vi "IECMemory.Tables2Array.vi"(5 "Timing Num":dbl[](array[numeric]), 9 "Logic":string[](array[string]), 11 "error in (no error)":errorcluster) -> (8 "MemData":dbl[][](array[numeric]), 15 "error out":errorcluster)   [LabVIEW 2014, in "IECMemory.lvlib"]
uses:
  IECMemory.lvlib
panel:
  in  "Channel":i32
  in  "Index":i32
  in  "Upper/Lower?":string
  out "Decomposed Logic Strings":string[][](array[string])
  out "Logic Strings Length":i32[](array[numeric])
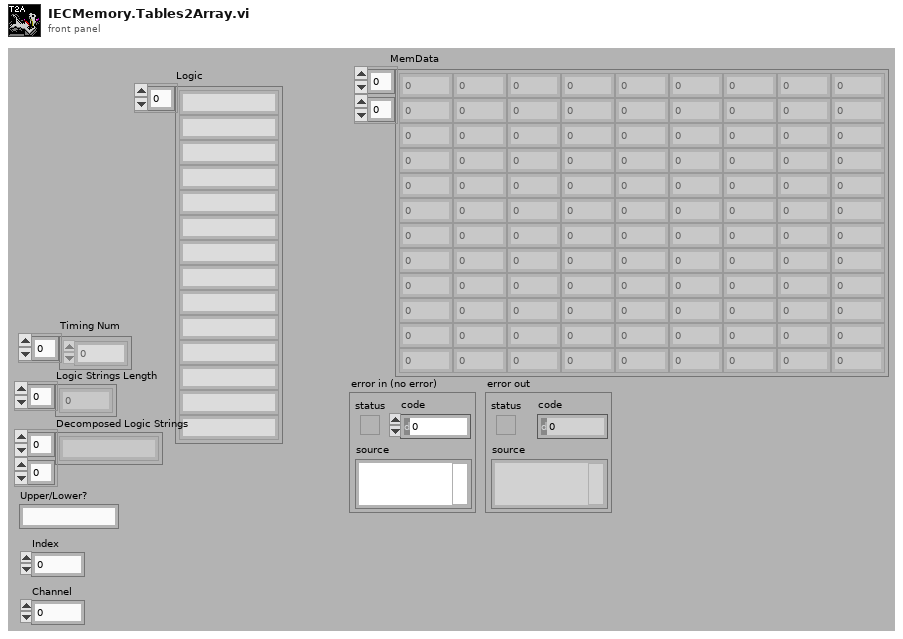
[diagram p1: front panel]
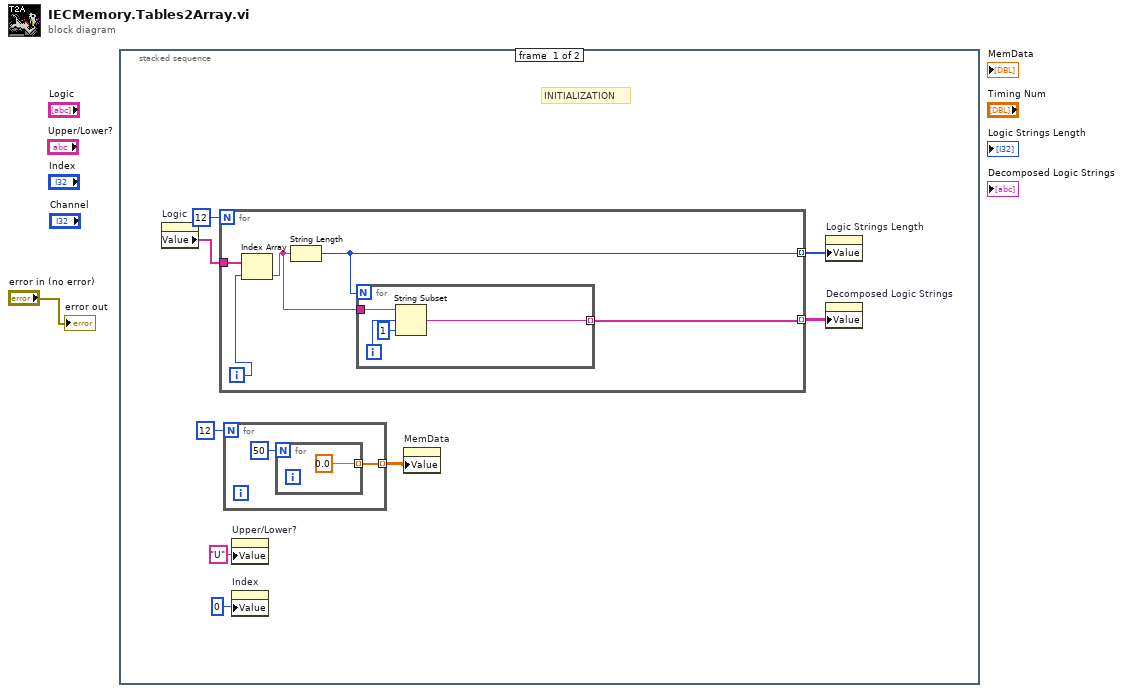
[diagram p0: block diagram]
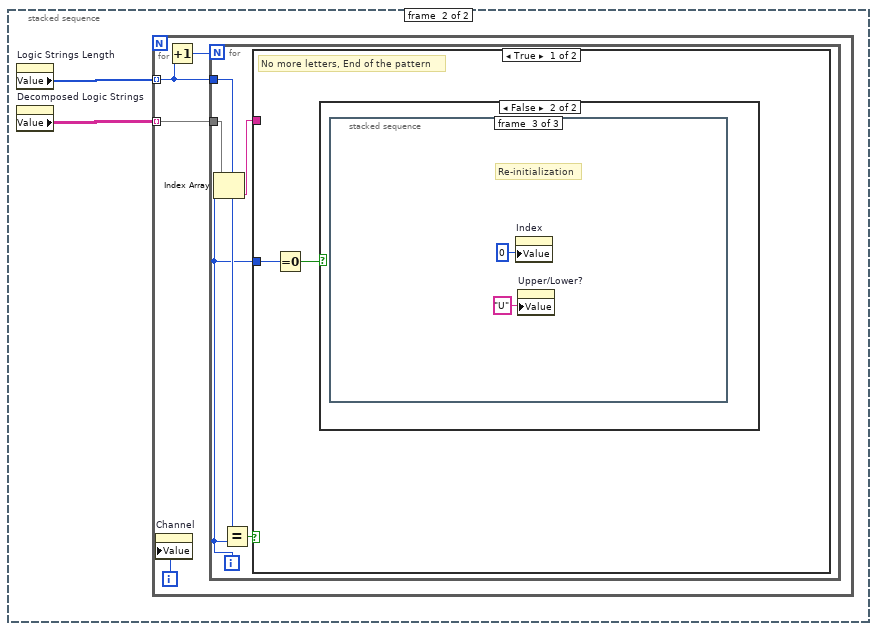
[diagram p2: hidden frame]
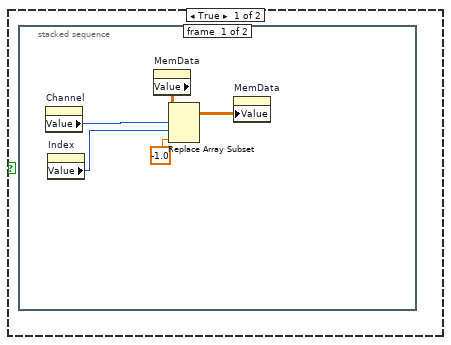
[diagram p3: hidden frame]
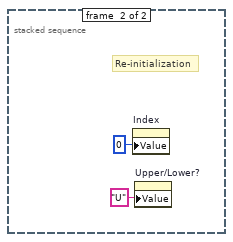
[diagram p4: hidden frame]
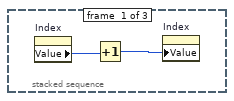
[diagram p5: hidden frame]
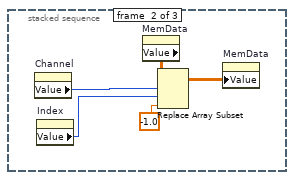
[diagram p6: hidden frame]
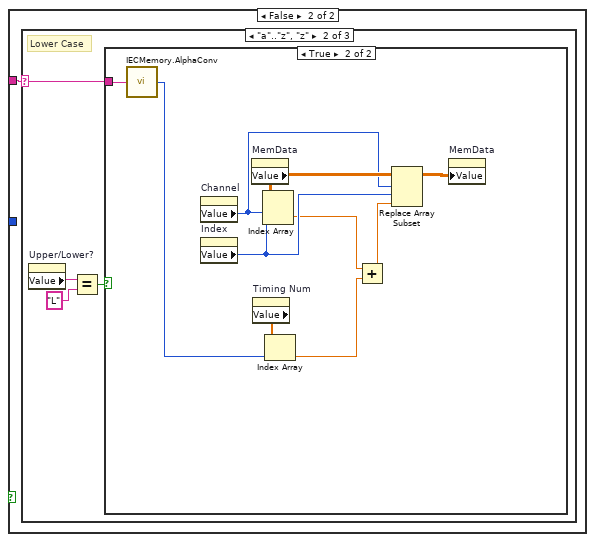
[diagram p7: hidden frame]
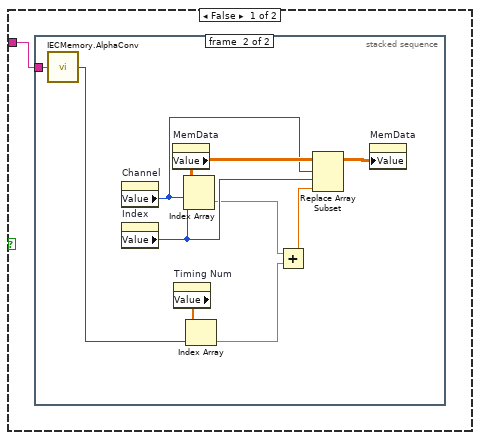
[diagram p9: hidden frame]
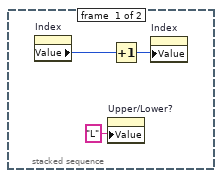
[diagram p10: hidden frame]
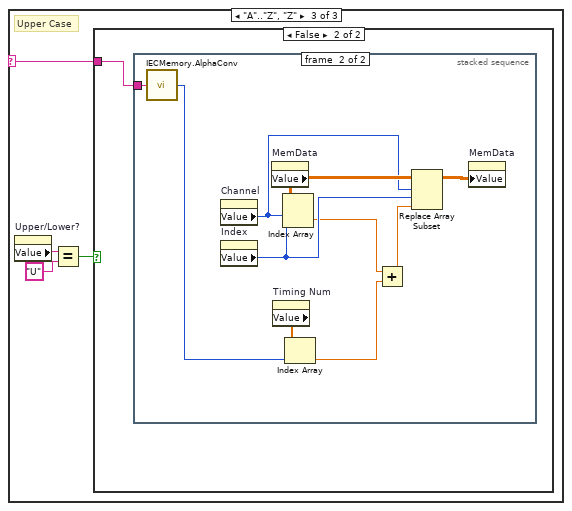
[diagram p11: hidden frame]
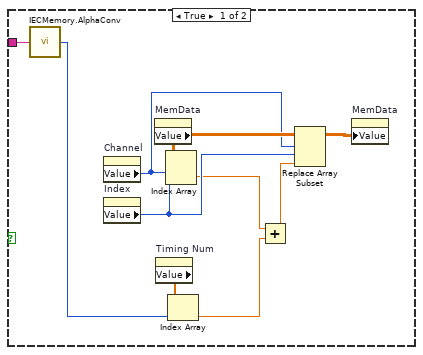
[diagram p12: hidden frame]
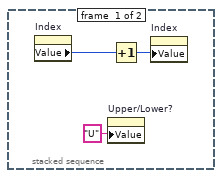
[diagram p13: hidden frame]
diagram:
  n1 = stacked-sequence {
    frame #0 {
      # "INITIALIZATION"
      n2 = property on="Logic" class="Arr (strict)"() -> ("Value"=w3:string[])  [unwired: 2 in, 2 out]
      n3 = for {
        N: 12 -> [_]
        tunnel: [w17] -> w9 mode=indexing
        tunnel: [w16] -> w8 mode=indexing
        tunnel: w3 -> [w14]
        i -> [w15]
        n4 = Index Array(array=w14, index=w15) -> (element=w13:string)
        n5 = String Length(string=w13) -> (length=w17:i32)
        n6 = for {
          N: w17 -> [_]
          tunnel: w13 -> [w21]
          tunnel: [w18] -> w16 mode=indexing
          i -> [w19]
          n7 = String Subset(string=w21, offset (0)=w19, length (rest)=1 ("length (rest)")) -> (substring=w18:string)
        }
      }
      n8 = for {
        N: 12 -> [_]
        tunnel: [w10] -> w6 mode=indexing
        n9 = for {
          N: 50 -> [_]
          tunnel: [0.0] -> w10 mode=indexing
        }
      }
      n10 = property on="Upper/Lower?" class="Str"("Value"="U" ("Upper/Lower?")) -> ()  [unwired: 2 in, 2 out]
      n11 = property on="Index" class="DigNum (strict)"("Value"=0 ("Index")) -> ()  [unwired: 2 in, 2 out]
      n12 = property on="MemData" class="Arr (strict)"("Value"=w6) -> ()  [unwired: 2 in, 2 out]
      n13 = property on="Logic Strings Length" class="Arr (strict)"("Value"=w9) -> ()  [unwired: 2 in, 2 out]
      n14 = property on="Decomposed Logic Strings" class="Arr (strict)"("Value"=w8) -> ()  [unwired: 2 in, 2 out]
    }
    frame #1 {
      n15 = property on="Logic Strings Length" class="Arr (strict)"() -> ("Value"=w22:i32[])  [unwired: 2 in, 2 out]
      n16 = property on="Decomposed Logic Strings" class="Arr (strict)"() -> ("Value"=w23:string[][])  [unwired: 2 in, 2 out]
      n17 = for {
        tunnel: w23 -> [w24] mode=indexing
        tunnel: w22 -> [w25] mode=indexing
        i -> [w27]
        n18 = property on="Channel" class="DigNum (strict)"("Value"=w27) -> ()  [unwired: 2 in, 2 out]
        n19 = Increment(x=w25) -> (x+1=w26:i32)
        n20 = for {
          N: w26 -> [_]
          tunnel: w25 -> [w32]
          tunnel: w24 -> [w30]
          i -> [w28]
          n21 = Index Array(array=w30, index=w28) -> (element=w29:string)
          n22 = Equal?(x=w32, y=w28) -> (x = y?=w31:bool)
          n23 = case shown="True" w31 {
            tunnel: w29 -> [_ w51]
            tunnel: w28 -> [w34 _]
            frame True {
              # "No more letters, End of the pattern"
              n24 = Equal To 0?(x=w34) -> (x = 0?=w33:bool)
              n25 = case shown="False" w33 {
                frame True {
                  n26 = stacked-sequence {
                    frame #0 {
                      n27 = property on="Channel" class="DigNum (strict)"() -> ("Value"=w37:i32)  [unwired: 2 in, 2 out]
                      n28 = property on="Index" class="DigNum (strict)"() -> ("Value"=w35:i32)  [unwired: 2 in, 2 out]
                      n29 = property on="MemData" class="Arr (strict)"() -> ("Value"=w39:dbl[][])  [unwired: 2 in, 2 out]
                      n30 = Replace Array Subset(array=w39, new element=-1.0, index (row)=w37, index (col)=w35) -> (w36:dbl[][])
                      n31 = property on="MemData" class="Arr (strict)"("Value"=w36) -> ()  [unwired: 2 in, 2 out]
                    }
                    frame #1 {
                      # "Re-initialization"
                      n32 = property on="Index" class="DigNum (strict)"("Value"=0 ("Index")) -> ()  [unwired: 2 in, 2 out]
                      n33 = property on="Upper/Lower?" class="Str"("Value"="U" ("Upper/Lower?")) -> ()  [unwired: 2 in, 2 out]
                    }
                  }
                }
                frame False {
                  n34 = stacked-sequence {
                    frame #0 {
                      n35 = property on="Index" class="DigNum (strict)"() -> ("Value"=w43:i32)  [unwired: 2 in, 2 out]
                      n36 = Increment(x=w43) -> (x+1=w42:i32)
                      n37 = property on="Index" class="DigNum (strict)"("Value"=w42) -> ()  [unwired: 2 in, 2 out]
                    }
                    frame #1 {
                      n38 = property on="Channel" class="DigNum (strict)"() -> ("Value"=w46:i32)  [unwired: 2 in, 2 out]
                      n39 = property on="Index" class="DigNum (strict)"() -> ("Value"=w44:i32)  [unwired: 2 in, 2 out]
                      n40 = property on="MemData" class="Arr (strict)"() -> ("Value"=w48:dbl[][])  [unwired: 2 in, 2 out]
                      n41 = Replace Array Subset(array=w48, new element=-1.0, index (row)=w46, index (col)=w44) -> (w45:dbl[][])
                      n42 = property on="MemData" class="Arr (strict)"("Value"=w45) -> ()  [unwired: 2 in, 2 out]
                    }
                    frame #2 {
                      # "Re-initialization"
                      n43 = property on="Index" class="DigNum (strict)"("Value"=0 ("Index")) -> ()  [unwired: 2 in, 2 out]
                      n44 = property on="Upper/Lower?" class="Str"("Value"="U" ("Upper/Lower?")) -> ()  [unwired: 2 in, 2 out]
                    }
                  }
                }
              }
            }
            frame False {
              n45 = case shown="\"a\"..\"z\", \"z\"" w51 {
                selector: w51 -> [_ w52 w80]
                frame "", "*", Default {
                  # "DO NOTHING"
                  # "Channel not in use"
                }
                frame "a".."z", "z" {
                  # "Lower Case"
                  n46 = property on="Upper/Lower?" class="Str"() -> ("Value"=w54:string)  [unwired: 2 in, 2 out]
                  n47 = Equal?(x=w54, y="L") -> (x = y?=w55:bool)
                  n48 = case shown="True" w55 {
                    tunnel: w52 -> [w56 w70]
                    frame False {
                      n49 = stacked-sequence {
                        tunnel: w56 -> [_ w69]
                        frame #0 {
                          n50 = property on="Index" class="DigNum (strict)"() -> ("Value"=w58:i32)  [unwired: 2 in, 2 out]
                          n51 = property on="Upper/Lower?" class="Str"("Value"="L" ("Upper/Lower?")) -> ()  [unwired: 2 in, 2 out]
                          n52 = Increment(x=w58) -> (x+1=w59:i32)
                          n53 = property on="Index" class="DigNum (strict)"("Value"=w59) -> ()  [unwired: 2 in, 2 out]
                        }
                        frame #1 {
                          n54 = call "IECMemory.AlphaConv.vi"("String"=w69) -> ("Numeric"=w64:i32)  [unwired: 14 in]
                          n55 = property on="Channel" class="DigNum (strict)"() -> ("Value"=w65:i32)  [unwired: 2 in, 2 out]
                          n56 = property on="Index" class="DigNum (strict)"() -> ("Value"=w66:i32)  [unwired: 2 in, 2 out]
                          n57 = property on="MemData" class="Arr (strict)"() -> ("Value"=w68:dbl[][])  [unwired: 2 in, 2 out]
                          n58 = property on="Timing Num" class="Arr (strict)"() -> ("Value"=w62:dbl[])  [unwired: 2 in, 2 out]
                          n59 = Index Array(array=w68, index (row)=w65, index (col)=w66) -> (element=w63:dbl)
                          n60 = Index Array(array=w62, index=w64) -> (element=w61:dbl)
                          n61 = Add(x=w63, y=w61) -> (x+y=w60:dbl)
                          n62 = Replace Array Subset(array=w68, new element=w60, index (row)=w65, index (col)=w66) -> (w67:dbl[][])
                          n63 = property on="MemData" class="Arr (strict)"("Value"=w67) -> ()  [unwired: 2 in, 2 out]
                        }
                      }
                    }
                    frame True {
                      n64 = call "IECMemory.AlphaConv.vi"("String"=w70) -> ("Numeric"=w75:i32)  [unwired: 14 in]
                      n65 = property on="Channel" class="DigNum (strict)"() -> ("Value"=w76:i32)  [unwired: 2 in, 2 out]
                      n66 = property on="Index" class="DigNum (strict)"() -> ("Value"=w77:i32)  [unwired: 2 in, 2 out]
                      n67 = property on="MemData" class="Arr (strict)"() -> ("Value"=w79:dbl[][])  [unwired: 2 in, 2 out]
                      n68 = property on="Timing Num" class="Arr (strict)"() -> ("Value"=w73:dbl[])  [unwired: 2 in, 2 out]
                      n69 = Index Array(array=w79, index (row)=w76, index (col)=w77) -> (element=w74:dbl)
                      n70 = Index Array(array=w73, index=w75) -> (element=w72:dbl)
                      n71 = Add(x=w74, y=w72) -> (x+y=w71:dbl)
                      n72 = Replace Array Subset(array=w79, new element=w71, index (row)=w76, index (col)=w77) -> (w78:dbl[][])
                      n73 = property on="MemData" class="Arr (strict)"("Value"=w78) -> ()  [unwired: 2 in, 2 out]
                    }
                  }
                }
                frame "A".."Z", "Z" {
                  # "Upper Case"
                  n74 = property on="Upper/Lower?" class="Str"() -> ("Value"=w83:string)  [unwired: 2 in, 2 out]
                  n75 = Equal?(x=w83, y="U") -> (x = y?=w81:bool)
                  n76 = case shown="False" w81 {
                    tunnel: w80 -> [w93 w94]
                    frame True {
                      n77 = call "IECMemory.AlphaConv.vi"("String"=w93) -> ("Numeric"=w88:i32)  [unwired: 14 in]
                      n78 = property on="Channel" class="DigNum (strict)"() -> ("Value"=w89:i32)  [unwired: 2 in, 2 out]
                      n79 = property on="Index" class="DigNum (strict)"() -> ("Value"=w90:i32)  [unwired: 2 in, 2 out]
                      n80 = property on="MemData" class="Arr (strict)"() -> ("Value"=w92:dbl[][])  [unwired: 2 in, 2 out]
                      n81 = property on="Timing Num" class="Arr (strict)"() -> ("Value"=w86:dbl[])  [unwired: 2 in, 2 out]
                      n82 = Index Array(array=w92, index (row)=w89, index (col)=w90) -> (element=w87:dbl)
                      n83 = Index Array(array=w86, index=w88) -> (element=w85:dbl)
                      n84 = Add(x=w87, y=w85) -> (x+y=w84:dbl)
                      n85 = Replace Array Subset(array=w92, new element=w84, index (row)=w89, index (col)=w90) -> (w91:dbl[][])
                      n86 = property on="MemData" class="Arr (strict)"("Value"=w91) -> ()  [unwired: 2 in, 2 out]
                    }
                    frame False {
                      n87 = stacked-sequence {
                        tunnel: w94 -> [_ w107]
                        frame #0 {
                          n88 = property on="Index" class="DigNum (strict)"() -> ("Value"=w96:i32)  [unwired: 2 in, 2 out]
                          n89 = property on="Upper/Lower?" class="Str"("Value"="U" ("Upper/Lower?")) -> ()  [unwired: 2 in, 2 out]
                          n90 = Increment(x=w96) -> (x+1=w97:i32)
                          n91 = property on="Index" class="DigNum (strict)"("Value"=w97) -> ()  [unwired: 2 in, 2 out]
                        }
                        frame #1 {
                          n92 = call "IECMemory.AlphaConv.vi"("String"=w107) -> ("Numeric"=w102:i32)  [unwired: 14 in]
                          n93 = property on="Channel" class="DigNum (strict)"() -> ("Value"=w103:i32)  [unwired: 2 in, 2 out]
                          n94 = property on="Index" class="DigNum (strict)"() -> ("Value"=w104:i32)  [unwired: 2 in, 2 out]
                          n95 = property on="MemData" class="Arr (strict)"() -> ("Value"=w106:dbl[][])  [unwired: 2 in, 2 out]
                          n96 = property on="Timing Num" class="Arr (strict)"() -> ("Value"=w100:dbl[])  [unwired: 2 in, 2 out]
                          n97 = Index Array(array=w106, index (row)=w103, index (col)=w104) -> (element=w101:dbl)
                          n98 = Index Array(array=w100, index=w102) -> (element=w99:dbl)
                          n99 = Add(x=w101, y=w99) -> (x+y=w98:dbl)
                          n100 = Replace Array Subset(array=w106, new element=w98, index (row)=w103, index (col)=w104) -> (w105:dbl[][])
                          n101 = property on="MemData" class="Arr (strict)"("Value"=w105) -> ()  [unwired: 2 in, 2 out]
                        }
                      }
                    }
                  }
                }
              }
            }
          }
        }
      }
    }
  }
  "error out" <- "error in (no error)"
